vi "Paskevits_Vladislav_read_t.vi"(8 "error in (no error)":errorcluster, 11 "String":string="t0=24.62 oC") -> (0 "error out":errorcluster, 3 "Temperature":dbl)   [LabVIEW 2018]
doc: "Use this template to build a VI to use as a subVI.\nTemperatureVI\nPract.Exers"
panel:
  out "offset past match":i32
  out "after substring":string
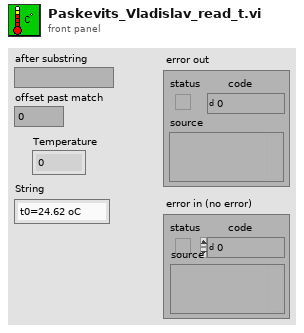
[diagram p1: front panel]
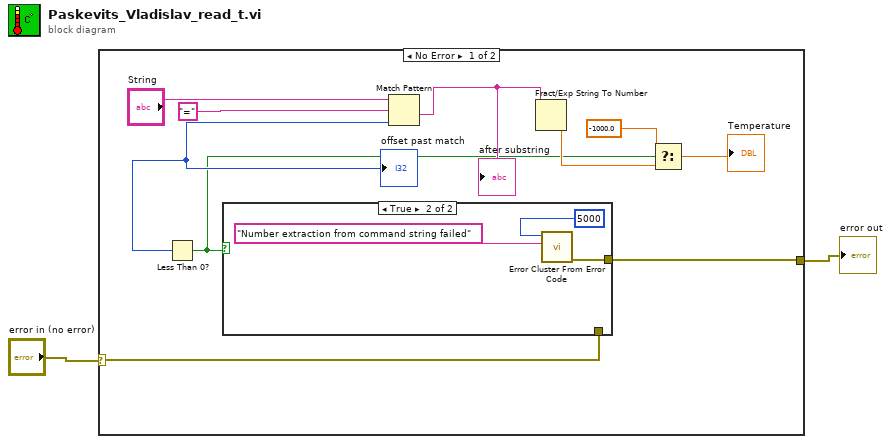
[diagram p0: block diagram]
diagram:
  n1 = case shown="No Error" "error in (no error)" {
    selector: "error in (no error)" -> [w7 w17]
    tunnel: [w8 w17] -> w1
    frame No Error {
      n2 = Match Pattern(string="String", regular expression="=" ("before substring")) -> (after substring=w10:string, offset past match=w9:i32)  [unwired: 1 in, 2 out]
      "after substring" <- w10
      "offset past match" <- w9
      n3 = Less Than 0?(x=w9) -> (x < 0?=w3:bool)
      n4 = case shown="True" w3 {
        tunnel: [w13 w14] -> w8
        tunnel: w7 -> [w13 _]
        frame False {
        }
        frame True {
          n5 = call <vilib>:"Error Cluster From Error Code.vi"("error message (\"\")"="Number extraction from command string failed" ("error message (\"\")"), "error code (0)"=5000) -> ("error out"=w14:errorcluster)  [unwired: 7 in]
        }
      }
      n6 = Fract/Exp String To Number(string=w10) -> (number=w4:dbl)  [unwired: 3 in, 1 out]
      n7 = Select(t=-1000.0, s=w3, f=w4) -> (s? t:f=→"Temperature":dbl)
    }
    frame Error {
    }
  }
  "error out" <- w1
